vi "Pseudo-random (Time-based) String.vi"(8 "Error In":errorcluster, 11 "Length (10)":u32=10) -> (0 "Error Out":errorcluster, 3 "result string":string)   [LabVIEW 2021, in "Strings.lvlib"]
uses:
  Strings.lvlib
  f784c936-4920-47f2-a9b9-59e3fd3c1f91.vi
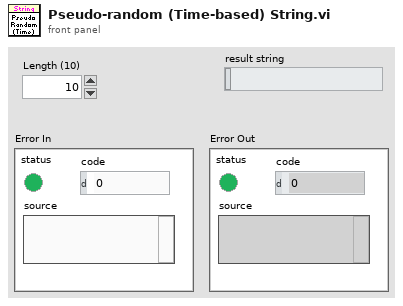
[diagram p1: front panel]
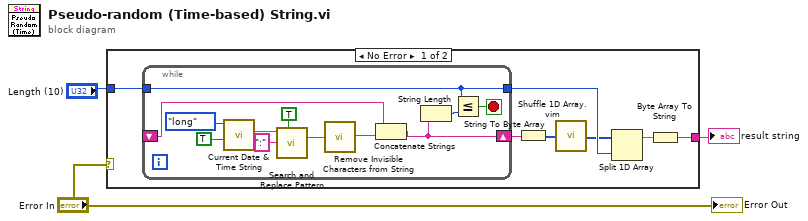
[diagram p0: block diagram]
diagram:
  n1 = case shown="No Error" "Error In" {
    tunnel: "Length (10)" -> [w10 _]
    tunnel: [w4 _] -> w1
    frame No Error {
      n2 = while {
        tunnel: w10 -> [w17]
        shift-right: [w15] -> w8
        shift-left: _ -> [w16]
        tunnel: [w17] -> w9
        stop <- w18 stop-if-true
        n3 = call "Current Date & Time String.vi"("want seconds? (T)"=TRUE, "date format (0)"=enum16{"short", "long", "abbreviated"}."long") -> ("time string"=w20:string)  [unwired: 7 in, 2 out]
        n4 = call <vilib>:"Search and Replace Pattern.vi"("string"=w20, "regular expression (\"\")"=":" ("regular expression (\"\")"), "replace all? (F)"=TRUE) -> ("result string"=w12:string)  [unwired: 2 in, 1 out]
        n5 = call "Remove Invisible Characters from String.vi"("String"=w12) -> ("result string"=w11:string)  [unwired: 3 in]
        n6 = Concatenate Strings(w16, w11) -> (w15:string)
        n7 = String Length(string=w15) -> (length=w19:i32)
        n8 = Less Or Equal?(x=w17, y=w19) -> (x <= y?=w18:bool)
      }
      n9 = String To Byte Array(string=w8) -> (unsigned byte array=w7:u8[])
      n10 = call "Shuffle 1D Array.vim"("array"=w7) -> ("shuffled array"=w6:u8[])  [unwired: 4 in]
      n11 = Split 1D Array(array=w6, index=w9) -> (first subarray=w5:u8[])  [unwired: 1 out]
      n12 = Byte Array To String(unsigned byte array=w5) -> (string=w4:string)
    }
    frame Error {
    }
  }
  "result string" <- w1
  "Error Out" <- "Error In"
